vi "AB_Engine_CreateVisitedVIsStructures.vi"(10 "paths":path[](array[path]), 11 "Build app instance":refnum<vi>) -> (1 "Visited VIs Hash":variant, 2 "Visited VIs Array":T1[](array[typedef]), 3 "Build app instance out":refnum<vi>)   [LabVIEW 2020]
uses:
  <vilib>/AppBuilder/Engine/AB_Engine_PathNode.ctl
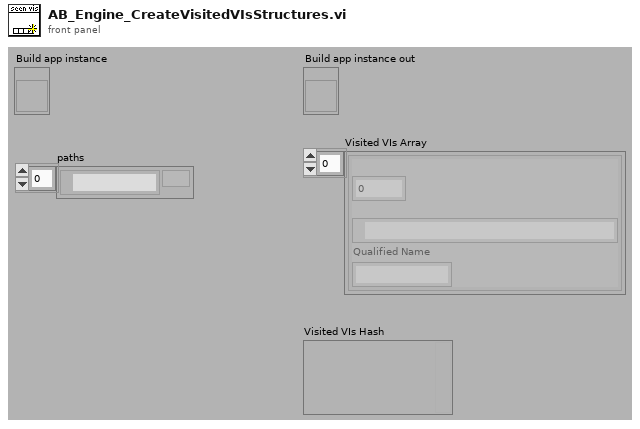
[diagram p1: front panel]
types:
  T1 = typedef "AB_Engine_PathNode.ctl" = cluster{"parent":i32, "path":path, "Qualified Name":string}
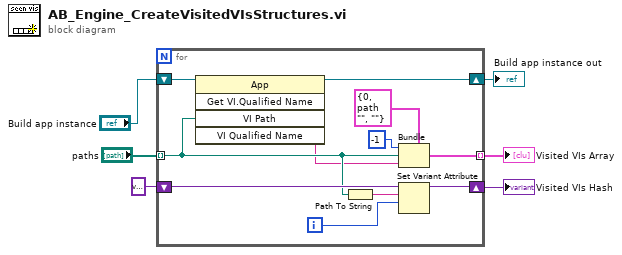
[diagram p0: block diagram]
diagram:
  n1 = for {
    tunnel: [w17] -> w3 mode=indexing
    tunnel: "paths" -> [w9] mode=indexing
    shift-right: [w14] -> w6
    shift-left: variant ("variant out") -> [w15]
    shift-right: [w7] -> w1
    shift-left: "Build app instance" -> [w10]
    i -> [w12]
    n2 = invoke class="App" method="Get VI.Qualified Name"(reference=w10, "VI Path"=w9) -> (reference out=w7:refnum<vi>, "VI Qualified Name"=w8:string)  [unwired: 3 in, 3 out]
    n3 = Path To String(path=w9) -> (string=w13:string)
    n4 = Bundle(cluster=T1 {"parent"=0, "path"=path "", "Qualified Name"=""} ("PathNode"), "parent"=-1, "path"=w9, "Qualified Name"=w8) -> (w17:T1)
    n5 = Set Variant Attribute(Variant=w15, name=w13, value=w12) -> (Variant out=w14:variant)  [unwired: 1 in, 2 out]
  }
  "Visited VIs Hash" <- w6
  "Visited VIs Array" <- w3
  "Build app instance out" <- w1
